vi "half (x + y) [I32].vi"(4 "y":i32, 5 "x":i32) -> (1 "(x+y)/2":i32)   [LabVIEW 2021, in "Math.lvlib"]
uses:
  Math.lvlib
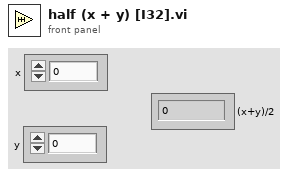
[diagram p1: front panel]
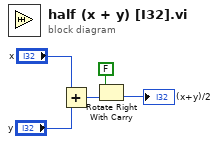
[diagram p0: block diagram]
diagram:
  n1 = Add(x="x", y="y") -> (x+y=w2:i32)
  n2 = Rotate Right With Carry(2:w2, 3:FALSE ("carry")) -> (0:→"(x+y)/2":i32)  [unwired: 1 out]
